vi "Read Initialised_.vi"(8 "error in (no error)":errorcluster, 11 "Singleton in":refnum<class "Singleton.lvclass">) -> (0 "error out":errorcluster, 2 "Initialised?":bool, 3 "Singleton out":refnum<class "Singleton.lvclass">)   [LabVIEW 2020, in "Singleton.lvlib" / "Singleton.lvclass"]
uses:
  Singleton.lvclass
  Singleton.lvclass/Singleton.ctl
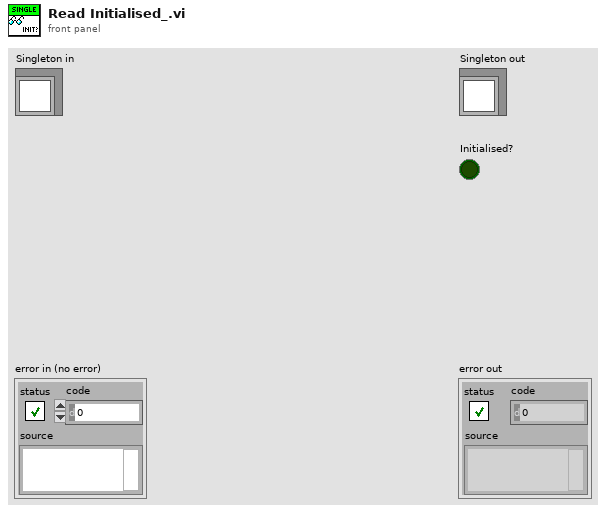
[diagram p1: front panel]
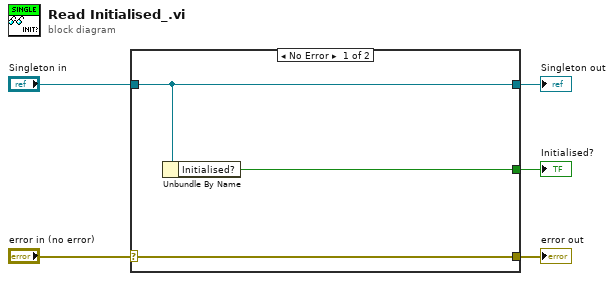
[diagram p0: block diagram]
diagram:
  n1 = case shown="No Error" "error in (no error)" {
    selector: "error in (no error)" -> [w8 w9]
    tunnel: [w8 w9] -> w4
    tunnel: [w7 w10] -> w2
    tunnel: "Singleton in" -> [w7 w10]
    tunnel: [w6 _] -> w1
    frame No Error {
      n2 = Unbundle By Name(w7) -> ("Initialised?"=w6:bool)
    }
    frame Error {
    }
  }
  "error out" <- w4
  "Singleton out" <- w2
  "Initialised?" <- w1
